vi "RTMain.Initialize.vi"(11 "Device Reference in":T1 format="%.0x") -> (0 "error out":errorcluster, 2 "Name":string, 3 "Parameters":T2 {"Settings"."Data Refs"."Write Refs" format="%.0x"; "Settings"."Data Refs"."Read Refs" format="%.0x"; "Settings"."Write Locations"."DataType" items=["Boolean"=1, "SByte"=2, "Byte"=3, "Int16"=4, "UInt16"=5, "Int32"=6, "UInt32"=7, "Int64"=8, "UInt64"=9, "Float"=10, "Double"=11, "String"=12, "DateTime"=13, "ByteString"=15, "Array of Boolean"=101, "Array of SByte"=102, "Array of Byte"=103, "Array of Int16"=104, "Array of UInt16"=105, "Array of Int32"=106, "Array of UInt32"=107, "Array of Int64"=108, "Array of UInt64"=109, "Array of Float"=110, "Array of Double"=111, "Array of String"=112, "Array of DateTime"=113, "Array of ByteString"=115]})   [LabVIEW 2019, in "OPC UA Client Addon Engine.lvlib"]
uses:
  OPC UA Client Addon Engine.lvlib
  Types/Poll.Parameters.ctl
  Addon Shared/Types/Compiled.Settings.ctl
  Addon Shared/Types/OPCConnection.Properties.ctl
  Addon Shared/Types/Poll.ListProperties.ctl
  Addon Shared/Types/Tag.WriteProperties.Info.ctl
  Addon Shared/Types/Tags.ReadWriteRefs.ctl
  <vilib>/NI VeriStand/Custom Device API/Data Reference.ctl
  <vilib>/NI VeriStand/Custom Device API/Custom Device Target Type.ctl
  <vilib>/NI VeriStand/Custom Device API/Custom Device Item Ref.ctl
  Addon Shared/SubVIs/Constants.vi
  <vilib>/NI VeriStand/Custom Device API/Get Item Property (Variant).vi
  <vilib>/Utility/SystemLogging/Write to System Log.vi
  <vilib>/NI VeriStand/Custom Device API/Custom Device API.lvlib
  Addon Shared/OPC UA Client Addon Shared.lvlib
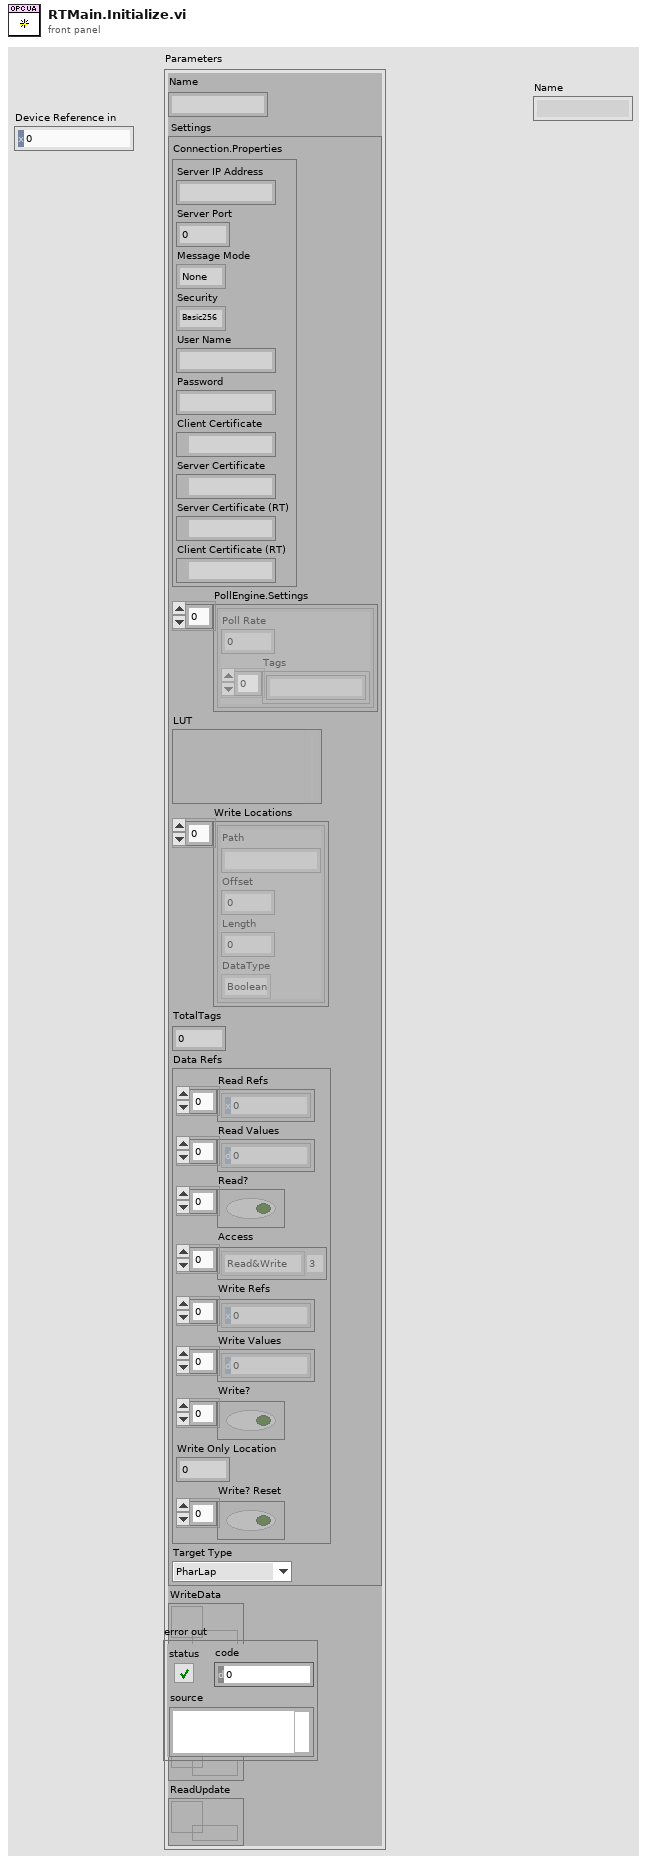
[diagram p1: front panel]
types:
  T1 = typedef "Custom Device API.lvlib/Custom Device Item Ref.ctl" = u64
  T2 = typedef "OPC UA Client Addon Engine.lvlib/Poll.Parameters.ctl" = cluster{"Name":string, "Settings":T3, "WriteData":refnum<k33>, "ReadData":refnum<k33>, "WriteUpdate":refnum<k33>, "ReadUpdate":refnum<k33>}
  T3 = typedef "OPC UA Client Addon Shared.lvlib/Compiled.Settings.ctl" = cluster{"Connection.Properties":T4, "PollEngine.Settings":T5[], "LUT":variant, "Write Locations":T6[], "TotalTags":u32, "Data Refs":T7, "Target Type":T9}
  T4 = typedef "OPC UA Client Addon Shared.lvlib/OPCConnection.Properties.ctl" = cluster{"Server IP Address":string, "Server Port":u16, "Message Mode":enum16{"None", "Sign", "Sign and Encrypt"}, "Security":enum16{"Basic256", "Basic128Rsa15"}, "User Name":string, "Password":string, "Client Certificate":path, "Server Certificate":path, "Server Certificate (RT)":path, "Client Certificate (RT)":path}
  T5 = typedef "OPC UA Client Addon Shared.lvlib/Poll.ListProperties.ctl" = cluster{"Poll Rate":dbl, "Tags":string[]}
  T6 = typedef "OPC UA Client Addon Shared.lvlib/Tag.WriteProperties.Info.ctl" = cluster{"Path":string, "Offset":i32, "Length":i32, "DataType":u32}
  T7 = typedef "OPC UA Client Addon Shared.lvlib/Tags.ReadWriteRefs.ctl" = cluster{"Read Refs":T8[], "Read Values":dbl[], "Read?":bool[], "Access":enum8{"Null", "Read", "Write", "Read&Write"}[], "Write Refs":T8[], "Write Values":dbl[], "Write?":bool[], "Write Only Location":u32, "Write? Reset":bool[]}
  T8 = typedef "Custom Device API.lvlib/Data Reference.ctl" = i32
  T9 = typedef "Custom Device API.lvlib/Custom Device Target Type.ctl" = enum16{"PharLap", "VxWorks", "Windows", "Linux_32_ARM", "Linux_x64"}
  T10 = cluster{"read mode":enum16{"polling", "blocking"}, "write mode":enum16{"polling", "blocking"}}
  T11 = typedef "Custom Device API.lvlib/Custom Device Item Info.ctl" = cluster{"Name":string, "Is Channel":bool, "GUID":string, "Is Waveform":bool}
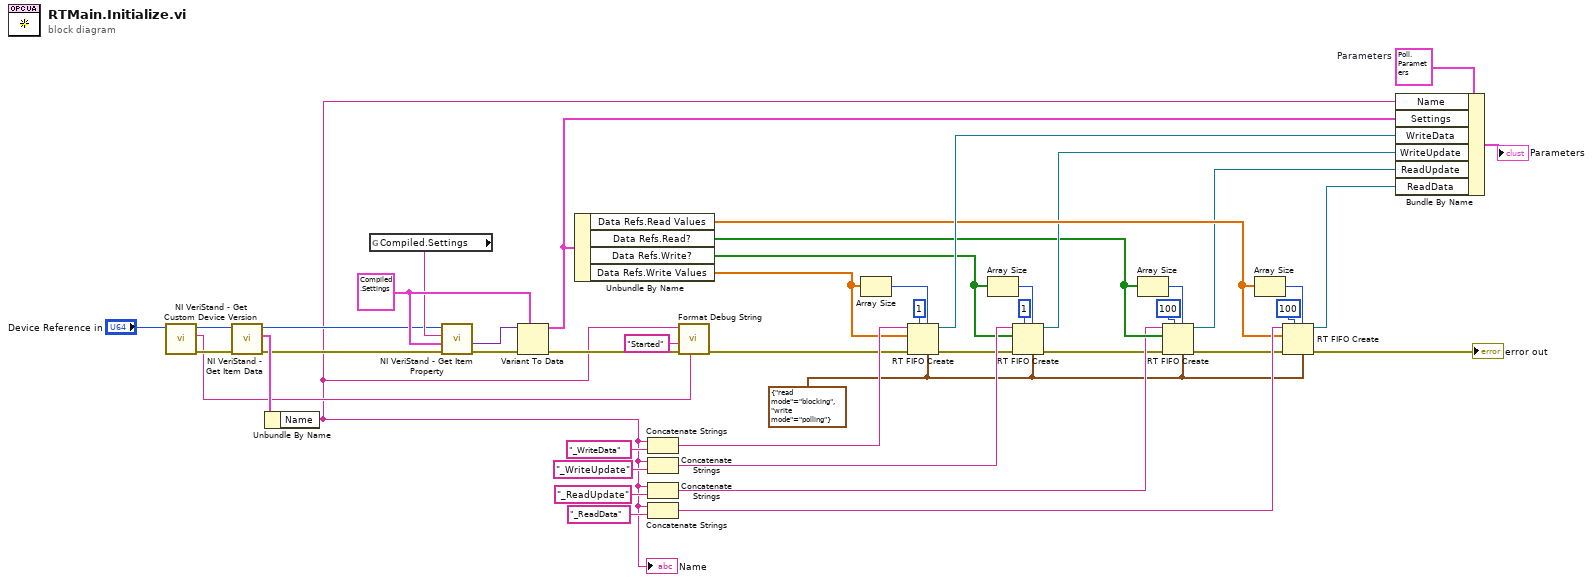
[diagram p0: block diagram]
diagram:
  w11 = T10 {"read mode"=enum."blocking", "write mode"=enum."polling"} ("r/w modes (polling,polling)")
  w45 = T2 {"Name"="", "Settings"={"Connection.Properties"={"Server IP Address"="", "Server Port"=0, "Message Mode"=enum."None", "Security"=enum."Basic256", "User Name"="", "Password"="", "Client Certificate"=path "", "Server Certificate"=path "", "Server Certificate (RT)"=path "", "Client Certificate (RT)"=path ""}, "PollEngine.Settings"=[], "LUT"=variant, "Write Locations"=[], "TotalTags"=0, "Data Refs"={"Read Refs"=[], "Read Values"=[], "Read?"=[], "Access"=[], "Write Refs"=[], "Write Values"=[], "Write?"=[], "Write Only Location"=0, "Write? Reset"=[]}, "Target Type"=enum."PharLap"}, "WriteData"=refnum, "ReadData"=refnum, "WriteUpdate"=refnum, "ReadUpdate"=refnum}  # Parameters
  w38 = T3 {"Connection.Properties"={"Server IP Address"="", "Server Port"=0, "Message Mode"=enum."None", "Security"=enum."Basic256", "User Name"="", "Password"="", "Client Certificate"=path "", "Server Certificate"=path "", "Server Certificate (RT)"=path "", "Client Certificate (RT)"=path ""}, "PollEngine.Settings"=[], "LUT"=variant, "Write Locations"=[], "TotalTags"=0, "Data Refs"={"Read Refs"=[], "Read Values"=[], "Read?"=[], "Access"=[], "Write Refs"=[], "Write Values"=[], "Write?"=[], "Write Only Location"=0, "Write? Reset"=[]}, "Target Type"=enum."PharLap"} ("Compiled.Settings")
  n1 = call <vilib>:"NI VeriStand - Get Custom Device Version.vi"("Device Ref in"="Device Reference in") -> ("error out"=w6:errorcluster, "Value"=w3:string, "Device Ref out"=w7:T1)  [unwired: 8 in]
  n2 = call <vilib>:"NI VeriStand - Get Item Data.vi"("error in (no error)"=w6, "Item Ref in"=w7) -> ("error out"=w10:errorcluster, "Item Info"=w39:T11, "Item Ref out"=w9:T1)  [unwired: 6 in, 1 out]
  n3 = Unbundle By Name(w39) -> ("Name"=w2:string)
  "Name" <- w2
  n4 = global read "Constants.vi" "Compiled.Settings"() -> (w37:string)
  n5 = call-poly <vilib>:"NI VeriStand - Get Item Property.vi"("error in (no error)"=w10, "Default Value"=w38, "Property Name"=w37, "Item Ref in"=w9) -> ("error out"=w35:errorcluster, "Value"=w36:variant)  [unwired: 4 in, 2 out]
  n6 = Variant To Data(error in=w35, type=w38, Variant=w36) -> (data=w34:T3, error out=w5:errorcluster)
  n7 = Unbundle By Name(w34) -> ("Data Refs.Read Values"=w33:dbl[], "Data Refs.Read?"=w28:bool[], "Data Refs.Write?"=w12:bool[], "Data Refs.Write Values"=w13:dbl[])
  n8 = Concatenate Strings(w2, "_WriteData" ("string")) -> (w42:string)
  n9 = Concatenate Strings(w2, "_WriteUpdate" ("string")) -> (w29:string)
  n10 = Concatenate Strings(w2, "_ReadUpdate" ("string")) -> (w26:string)
  n11 = Concatenate Strings(w2, "_ReadData" ("string")) -> (w43:string)
  n12 = call "Format Debug String.vi"("Version"=w3, "error in (no error)"=w5, "State"="Started", "Name"=w2) -> ("error out"=w4:errorcluster)  [unwired: 7 in]
  n13 = Array Size(array=w13) -> (size(s)=w23:i32)
  n14 = RT FIFO Create(0:w42, 1:w13, 3:w4, 4:u32 1 ("size (10)"), 6:w23, 7:w11) -> (8:w46:refnum<k33>, 11:w20:errorcluster)  [unwired: 2 in, 1 out]
  n15 = Array Size(array=w12) -> (size(s)=w19:i32)
  n16 = RT FIFO Create(0:w29, 1:w12, 3:w20, 4:u32 1 ("size (10)"), 6:w19, 7:w11) -> (8:w31:refnum<k33>, 11:w14:errorcluster)  [unwired: 2 in, 1 out]
  n17 = Array Size(array=w28) -> (size(s)=w16:i32)
  n18 = RT FIFO Create(0:w26, 1:w28, 3:w14, 4:u32 100 ("size (10)"), 6:w16, 7:w11) -> (8:w25:refnum<k33>, 11:w15:errorcluster)  [unwired: 2 in, 1 out]
  n19 = Array Size(array=w33) -> (size(s)=w22:i32)
  n20 = RT FIFO Create(0:w43, 1:w33, 3:w15, 4:u32 100 ("size (10)"), 6:w22, 7:w11) -> (8:w32:refnum<k33>, 11:→"error out":errorcluster)  [unwired: 2 in, 1 out]
  n21 = Bundle By Name(cluster=w45, "Name"=w2, "Settings"=w34, "WriteData"=w46, "WriteUpdate"=w31, "ReadUpdate"=w25, "ReadData"=w32) -> (→"Parameters":T2)
